vi "swap-Motor-v2.vi"(7 "Refnum in M3":refnum<k7>, 8 "error in (no error)":errorcluster, 9 "Swap motor":bool, 10 "Refnum in M2":refnum<k7>, 11 "Refnum in M1":refnum<k7>) -> (0 "error out":errorcluster)   [LabVIEW 2021]
doc: "This VI swap Motors X-->Y | Y--> X\n\nAndré Romero - 2023\nandretec@ifsc.usp.br\nIFSC - USP"
uses:
  Global Motors.vi
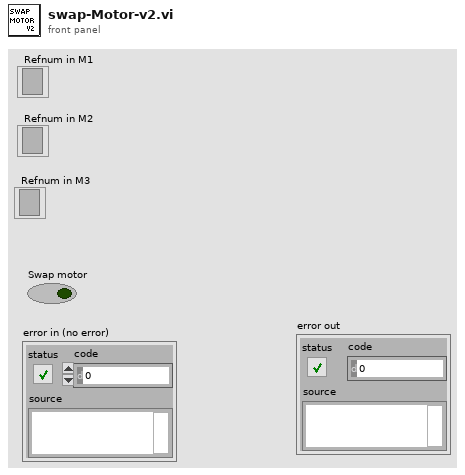
[diagram p1: front panel]
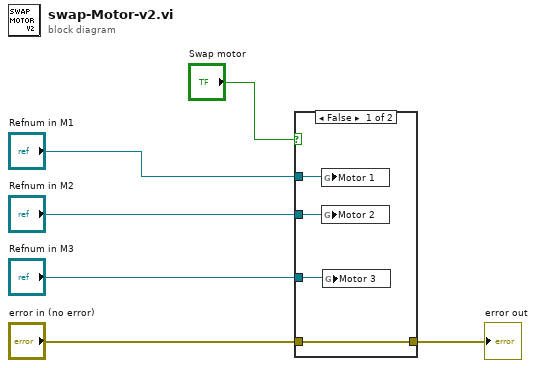
[diagram p0: block diagram]
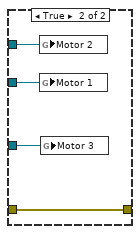
[diagram p2: hidden frame]
diagram:
  n1 = case shown="False" "Swap motor" {
    tunnel: "Refnum in M1" -> [w9 w13]
    tunnel: "Refnum in M2" -> [w10 w14]
    tunnel: "error in (no error)" -> [w8 w12]
    tunnel: [w8 w12] -> w6
    tunnel: "Refnum in M3" -> [w7 w11]
    frame False {
      n2 = global write "Global Motors.vi" "Motor 1"(w9) -> ()
      n3 = global write "Global Motors.vi" "Motor 2"(w10) -> ()
      n4 = global write "Global Motors.vi" "Motor 3"(w7) -> ()
    }
    frame True {
      n5 = global write "Global Motors.vi" "Motor 2"(w13) -> ()
      n6 = global write "Global Motors.vi" "Motor 1"(w14) -> ()
      n7 = global write "Global Motors.vi" "Motor 3"(w11) -> ()
    }
  }
  "error out" <- w6
